vi "realTimeMeasure.vi"() -> ()   [LabVIEW 2012]
doc: "This VI will continuously monitor the serial port and extract the temperature reading from the received string. This is stored in an array and displayed on the Graph. Press STOP to close the serial port and end the program.\n\nThis program is designed to work with the May 2009 version of the Arduino Temperature program which sends a header, the raw A/D value and the temperature as a float text value.\n\nSelect the appropriate COM port before running this VI. Leave the other serial port settings at their default values (9600, 8, none, 1.0, none)."
uses:
  <vilib>/Instr/_visa.llb/VISA Configure Serial Port (Instr).vi
panel:
  out "serial repsonse":string
  out "CurTemp":dbl caption="Current Value"
  out "ADC Graph":dbl[](graph)
  in  "VISA resource name":refnum<visa-resource-name>="COM3"
  in  "baud rate (9600)":u32=9600
  in  "data bits (8)":u16=8 min=5 max=8 step=1
  in  "stop bits (10: 1 bit)":u16(ring)=10 items=["1.0"=10, "1.5"=15, "2.0"=20]
  in  "flow control (0:none)":u16(ring) items=["None", "XON/XOFF", "RTS/CTS", "XON/XOFF & RTS/CTS", "DTR/DSR", "XON/XOFF & DTR/DSR"]
  in  "parity (0:none)":enum16{"None", "Odd", "Even", "Mark", "Space"}(ring)
  in  "stop":bool
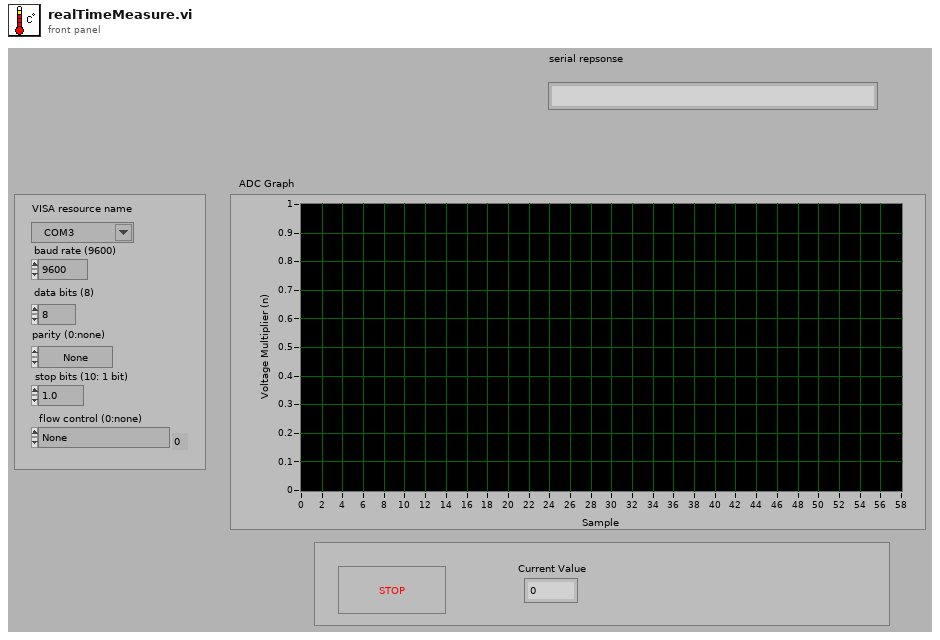
[diagram p1: front panel]
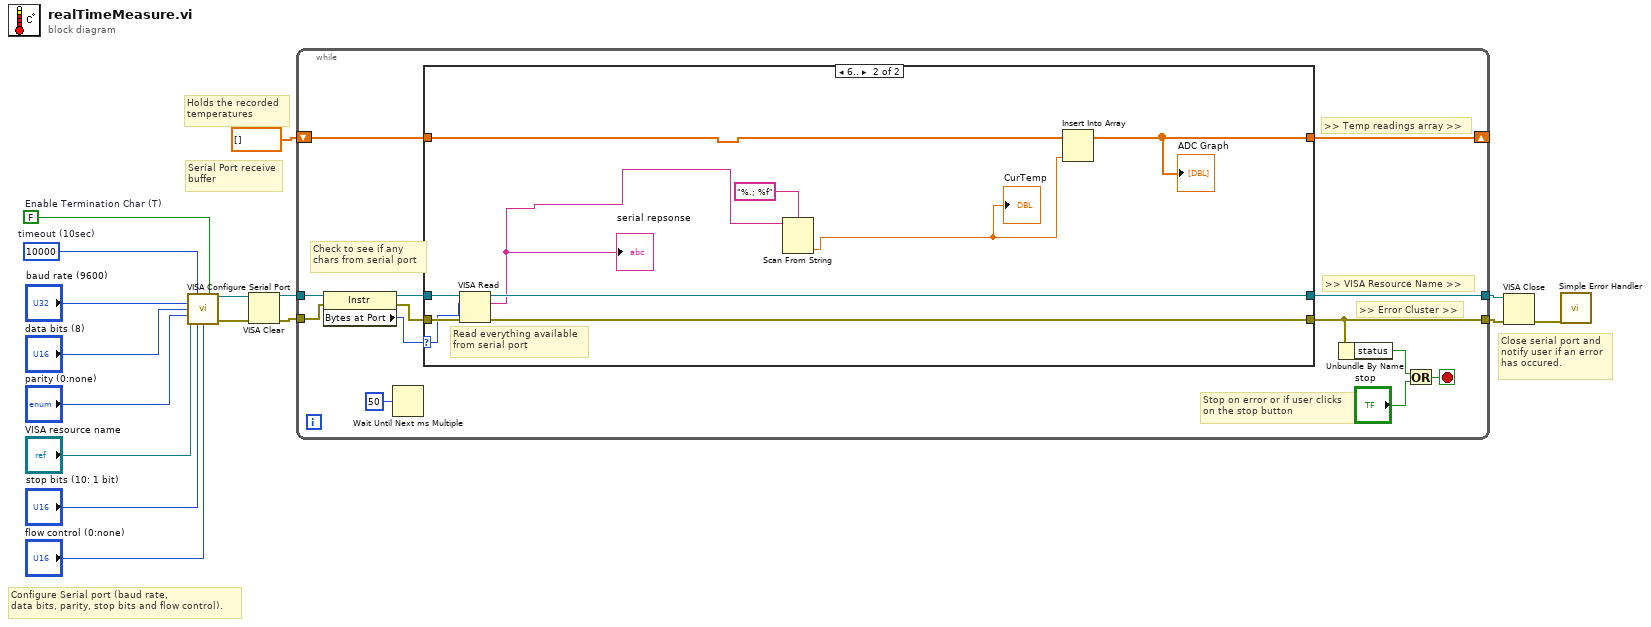
[diagram p0: block diagram]
diagram:
  w12 = FALSE  # Enable Termination Char (T)
  w13 = u32 10000  # timeout (10sec)
  # "Close serial port and\nnotify user if an error\nhas occured."
  # "Serial Port receive\nbuffer"
  # "Holds the recorded\ntemperatures"
  # "Configure Serial port (baud rate,\ndata bits, parity, stop bits and flow control)."
  n1 = call-poly "VISA Configure Serial Port"("VISA resource name"="VISA resource name", "timeout (10sec)"=w13, "Enable Termination\nChar (T)"=w12, "baud rate (9600)"="baud rate (9600)", "data bits (8)"="data bits (8)", "parity (0:none)"="parity (0:none)", "stop bits (10: 1 bit)"="stop bits (10: 1 bit)", "flow control (0:none)"="flow control (0:none)") -> ("VISA resource name out"=w10:refnum<visa-resource-name>, "error out"=w11:errorcluster)  [unwired: 6 in]
  n2 = VISA Clear(VISA resource name=w10, error in (no error)=w11) -> (VISA resource name out=w9:refnum<visa-resource-name>, error out=w8:errorcluster)
  n3 = while {
    tunnel: [w23] -> w16
    tunnel: [w29] -> w15
    tunnel: w9 -> [w26]
    tunnel: w8 -> [w25]
    shift-right: [w19] -> _
    shift-left: dbl[] [] -> [w18]
    stop <- w22 stop-if-true
    # "Stop on error or if user clicks \non the stop button"
    # ">> Error Cluster >>"
    # ">> VISA Resource Name >>"
    # ">> Temp readings array >>"
    # "Check to see if any\nchars from serial port"
    n4 = property class="Instr"(reference=w26, error in=w25) -> (reference out=w28:refnum<visa-resource-name>, error out=w27:errorcluster, "Bytes at Port"=w17:u32)
    n5 = Wait Until Next ms Multiple(millisecond multiple=u32 50) -> ()  [unwired: 1 out]
    n6 = case shown="6.." w17 {
      selector: w17 -> [_ w33]
      tunnel: [w31 w42] -> w23
      tunnel: [w32 w41] -> w29
      tunnel: w28 -> [w32 w40]
      tunnel: w27 -> [w31 w39]
      tunnel: [w30 w35] -> w19
      tunnel: w18 -> [w30 w36]
      frame 0, Default {
        # "No data in from serial port - Nothing to do."
      }
      frame 6.. {
        # "Read everything available\nfrom serial port"
        n7 = VISA Read(VISA resource name=w40, byte count=w33, error in (no error)=w39) -> (VISA resource name out=w41:refnum<visa-resource-name>, read buffer=w34:string, error out=w42:errorcluster)  [unwired: 1 out]
        "serial repsonse" <- w34
        n8 = Scan From String(format string="%.; %f", input string=w34) -> (output 1=w37:dbl)  [unwired: 3 in, 3 out]
        "CurTemp" <- w37
        n9 = Insert Into Array(array=w36, new element=w37) -> (w35:dbl[])  [unwired: 1 in]
        "ADC Graph" <- w35
      }
    }
    n10 = Unbundle By Name(w23) -> ("status"=w21:bool)
    n11 = Or(x=w21, y="stop") -> (x .or. y?=w22:bool)
  }
  n12 = VISA Close(VISA resource name=w15, error in (no error)=w16) -> (error out=w14:errorcluster)
  n13 = call <vilib>:"Simple Error Handler.vi"("error in (no error)"=w14) -> ()  [unwired: 4 in, 5 out]
